vi "AuxSensor_CAL 2016.vi"(6 "Sensor Cluster":T1, 7 "Array in":refnum<k24>[](array[refnum]), 8 "error in (no error)":errorcluster, 9 "Descriptions":string[](array[string]), 11 "Aux Sensor":i32) -> (0 "error out":errorcluster, 2 "Aux Sensor\nOffset (unit/V)":dbl format="%.4f", 3 "Aux Sensor\nSlope (unit/V)":dbl format="%.4f", 4 "Sensor Cluster 2":T1, 5 "Array out":refnum<k24>[](array[refnum]))   [LabVIEW 2016]
uses:
  C:/Cascade-lv16-64/builds/Waterloo Main Program/cascade/data/ULx_LV.dll
  builds/Waterloo Main Program/cascade/data/ULx_LV.dll
  controls/MCC DAQ Readings.ctl
panel:
  out "Aux Sensor\nVoltage 2 (V)":dbl format="%.4f"
  in  "Aux Sensor\nPhysical Parameter 2":dbl format="%.4f"
  in  "Aux Sensor\nPhysical Parameter 1":dbl format="%.4f"
  out "delta Parameter":dbl
  out "Aux Sensor\nVoltage 1 (V)":dbl format="%.4f"
  in  "stop":bool
  in  "start":bool
  # "AUXILLIARY SENSOR CALIBRATION"
  # "Enter Value for Physical Parameter Calibration Standard at Point 1.  Press start."
  # "Enter Value for Physical Parameter Calibration Standard at Point 2.  Press stop"
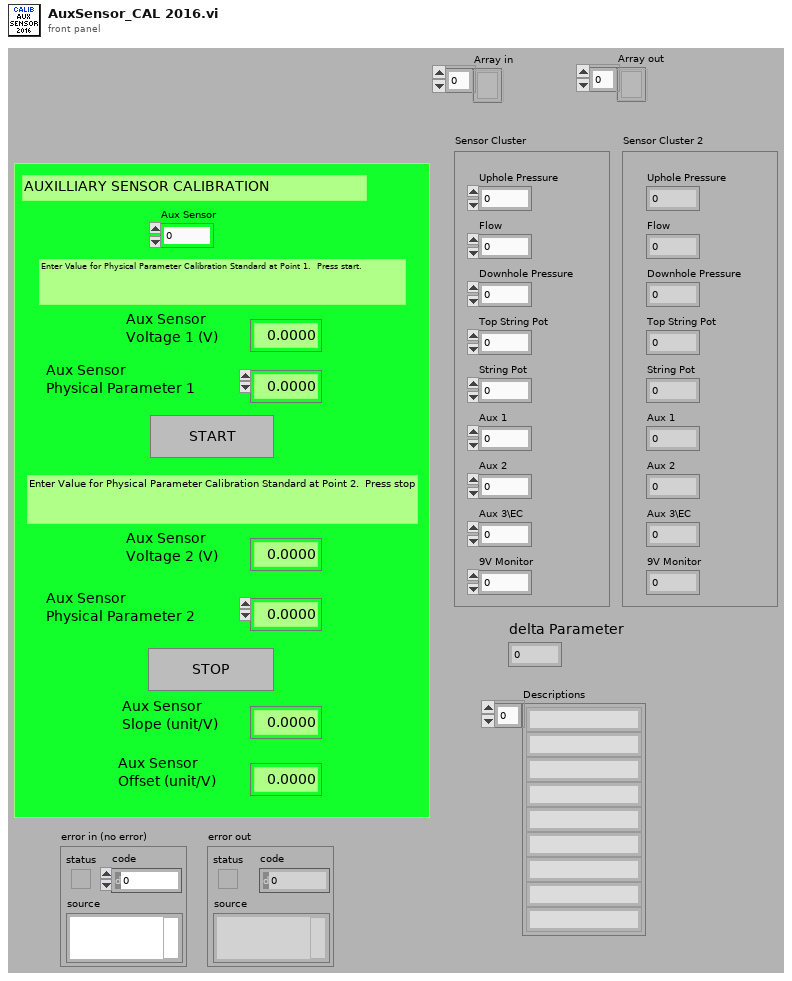
[diagram p1: front panel]
types:
  T1 = typedef "MCC DAQ Readings.ctl" = cluster{"Uphole Pressure":dbl, "Flow":dbl, "Downhole Pressure":dbl, "Top String Pot":dbl, "String Pot":dbl, "Aux 1":dbl, "Aux 2":dbl, "Aux 3\\EC":dbl, "9V Monitor":dbl}
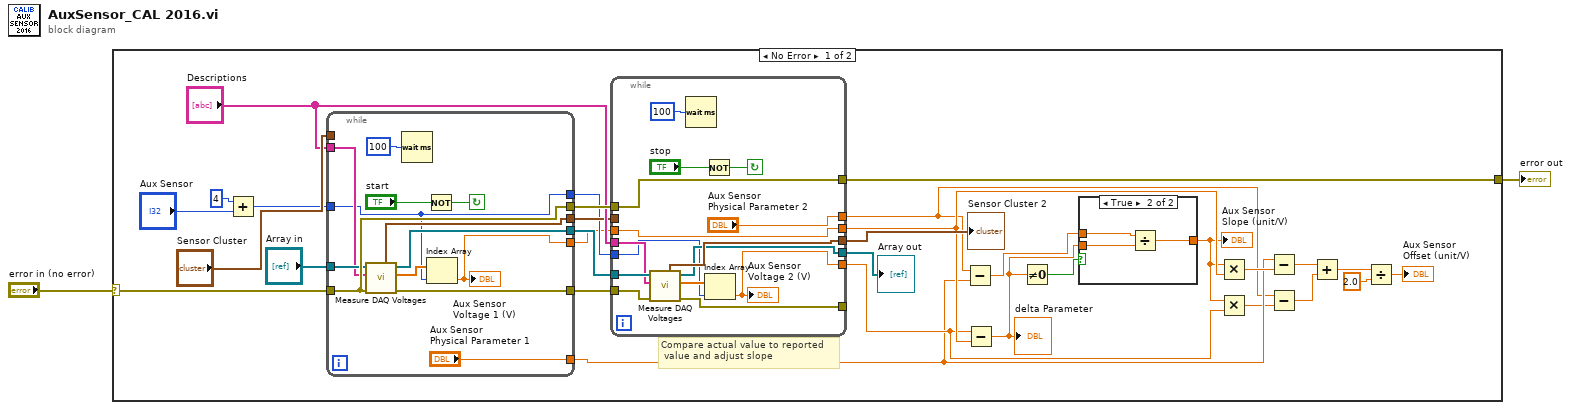
[diagram p0: block diagram]
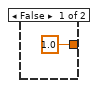
[diagram p2: hidden frame]
diagram:
  n1 = case shown="No Error" "error in (no error)" {
    selector: "error in (no error)" -> [w33 w66]
    tunnel: [w31 w66] -> w2
    frame No Error {
      # "Compare actual value to reported\n value and adjust slope"
      n2 = Add(x=4, y="Aux Sensor") -> (x+y=w18:i32)
      n3 = while {
        tunnel: [w47] -> w32
        tunnel: w33 -> [w47]
        tunnel: "Array in" -> [w46]
        tunnel: "Sensor Cluster" -> [_]
        tunnel: "Descriptions" -> [w43]
        tunnel: [w44] -> w25
        tunnel: [w45] -> w27
        tunnel: w18 -> [w40]
        tunnel: [w42] -> w21
        tunnel: [w40] -> w17
        tunnel: [w39] -> w16
        tunnel: ["Aux Sensor\nPhysical Parameter 1"] -> w10
        stop <- w49 continue-if-true
        n4 = call "Measure DAQ Voltages.vi"("error in (no error)"=w47, "Descriptions"=w43, "Array in"=w46) -> ("error in (no error) 2"=w42:errorcluster, "Raw Voltages"=w41:dbl[], "Array out"=w45:refnum<k24>[], "Sensor Cluster"=w44:T1)  [unwired: 5 in]
        n5 = Wait (ms)(milliseconds to wait=u32 100) -> ()  [unwired: 1 out]
        n6 = Not(x="start") -> (.not. x?=w49:bool)
        n7 = Index Array(array=w41, index=w40) -> (element=w39:dbl)
        "Aux Sensor\nVoltage 1 (V)" <- w39
      }
      n8 = while {
        tunnel: [w52] -> w14
        tunnel: [w53] -> w12
        tunnel: w32 -> [w63]
        tunnel: [w63] -> w31
        tunnel: "Descriptions" -> [w56]
        tunnel: w27 -> [w57]
        tunnel: [w58] -> w26
        tunnel: w25 -> [_]
        tunnel: [w59] -> w24
        tunnel: w21 -> [w61]
        tunnel: [w60] -> _
        tunnel: w17 -> [w54]
        tunnel: w16 -> [w52]
        tunnel: ["Aux Sensor\nPhysical Parameter 2"] -> w8
        stop <- w65 continue-if-true
        n9 = call "Measure DAQ Voltages.vi"("error in (no error)"=w61, "Descriptions"=w56, "Array in"=w57) -> ("error in (no error) 2"=w60:errorcluster, "Raw Voltages"=w55:dbl[], "Array out"=w58:refnum<k24>[], "Sensor Cluster"=w59:T1)  [unwired: 5 in]
        n10 = Wait (ms)(milliseconds to wait=u32 100) -> ()  [unwired: 1 out]
        n11 = Not(x="stop") -> (.not. x?=w65:bool)
        n12 = Index Array(array=w55, index=w54) -> (element=w53:dbl)
        "Aux Sensor\nVoltage 2 (V)" <- w53
      }
      "Sensor Cluster 2" <- w24
      "Array out" <- w26
      n13 = Subtract(x=w8, y=w10) -> (x-y=w15:dbl)
      n14 = Subtract(x=w12, y=w14) -> (x-y=w23:dbl)
      "delta Parameter" <- w23
      n15 = Not Equal To 0?(x=w23) -> (x != 0?=w22:bool)
      n16 = case shown="True" w22 {
        tunnel: w15 -> [_ w36]
        tunnel: [1.0 w35] -> w13
        tunnel: w23 -> [_ w37]
        frame False {
        }
        frame True {
          n17 = Divide(x=w36, y=w37) -> (x/y=w35:dbl)
        }
      }
      "Aux Sensor\nSlope (unit/V)" <- w13
      n18 = Multiply(x=w13, y=w14) -> (x*y=w11:dbl)
      n19 = Multiply(x=w13, y=w12) -> (x*y=w9:dbl)
      n20 = Subtract(x=w10, y=w11) -> (x-y=w7:dbl)
      n21 = Subtract(x=w8, y=w9) -> (x-y=w6:dbl)
      n22 = Add(x=w7, y=w6) -> (x+y=w5:dbl)
      n23 = Divide(x=w5, y=2.0) -> (x/y=→"Aux Sensor\nOffset (unit/V)":dbl)
    }
    frame Error {
    }
  }
  "error out" <- w2
